vi "ActionSCPICommand.vi"(8 "error in (no error)":errorcluster, 9 "DigitalOuts":T1, 10 "Analogs":T2, 11 "SCPI":string) -> (0 "error out":errorcluster, 3 "OutputMessage":string)   [LabVIEW 2022 SP3]
uses:
  Controls/Analogs.ctl
  Controls/DigitalOuts.ctl
  Controls/DisplayQCommand.ctl
  Controls/DisplayMessage.ctl
  <vilib>/Utility/error.llb/Trim Whitespace One-Sided.vi
  Globals/HandsOnGlobals.vi
panel:
  # "Output"
  # "Input"
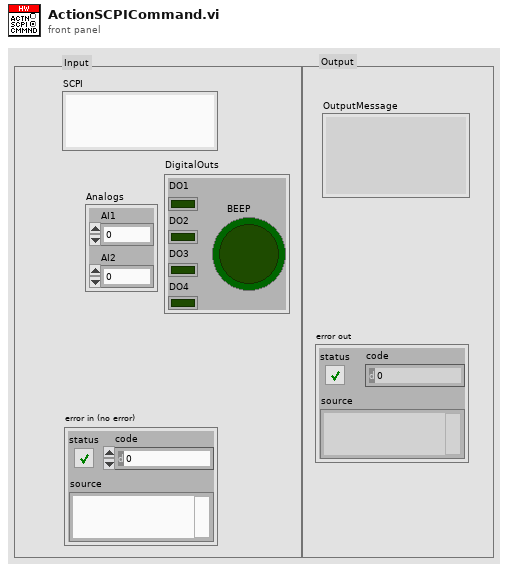
[diagram p1: front panel]
types:
  T1 = typedef "DigitalOuts.ctl" = cluster{"DO1":bool, "DO2":bool, "DO3":bool, "DO4":bool, "BEEP":bool}
  T2 = typedef "Analogs.ctl" = cluster{"AI1":u16, "AI2":u16}
  T3 = typedef "DisplayMessage.ctl" = enum16{"No Message - Ignore", "Display Message", "Set Tab", "Set Status", "Add Error Message", "Clear Error History", "Generate Error", "Set Idling Display", "Set Running Display", "Set DO1", "Set DO2", "Set DO3", "Set DO4", "Set AI1", "Set BEEP", "Update SCPI Return", "Clear SCPI", "Reset Screen", "Set PWM Duty", "Set PWM Freq", "Stop"}
  T4 = typedef "DisplayQCommand.ctl" = enum16{"No Command - Error", "Initialise", "Get Q Reference", "Add Item to Bottom", "Add Item to Top", "Flush Q", "Dequeue", "Peek Next Element", "Close"}
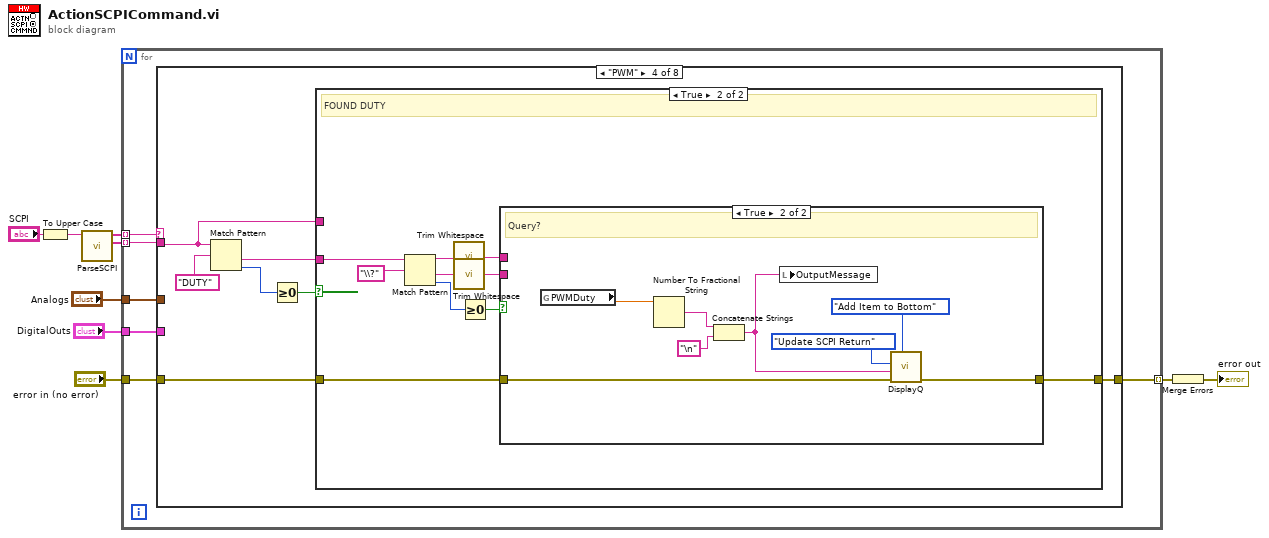
[diagram p0: block diagram]
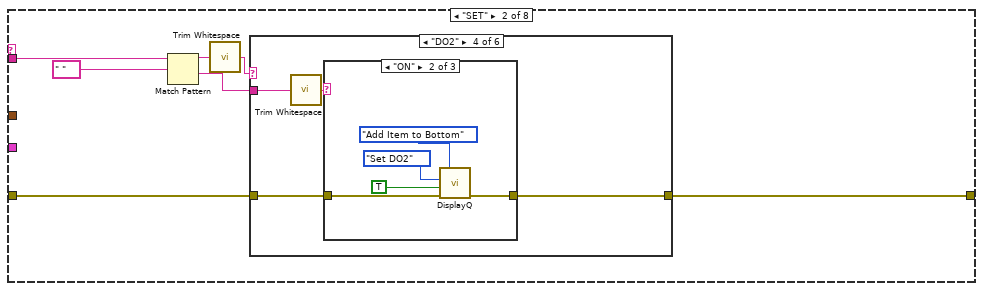
[diagram p3: hidden frame]
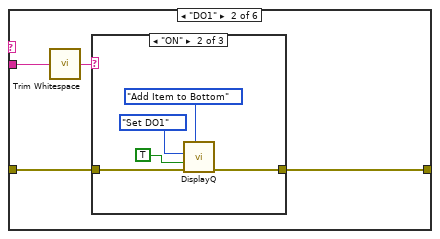
[diagram p5: hidden frame]
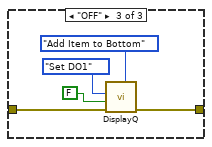
[diagram p7: hidden frame]
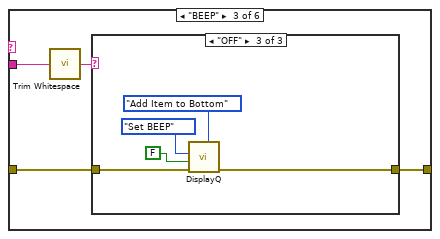
[diagram p8: hidden frame]
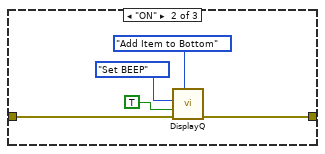
[diagram p10: hidden frame]
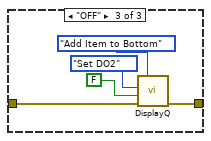
[diagram p12: hidden frame]
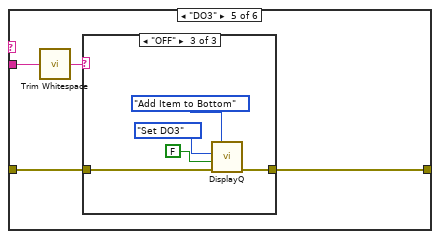
[diagram p13: hidden frame]
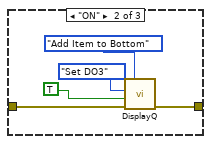
[diagram p15: hidden frame]
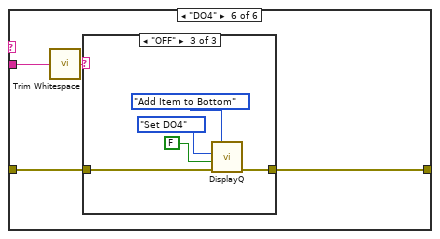
[diagram p16: hidden frame]
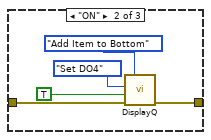
[diagram p18: hidden frame]
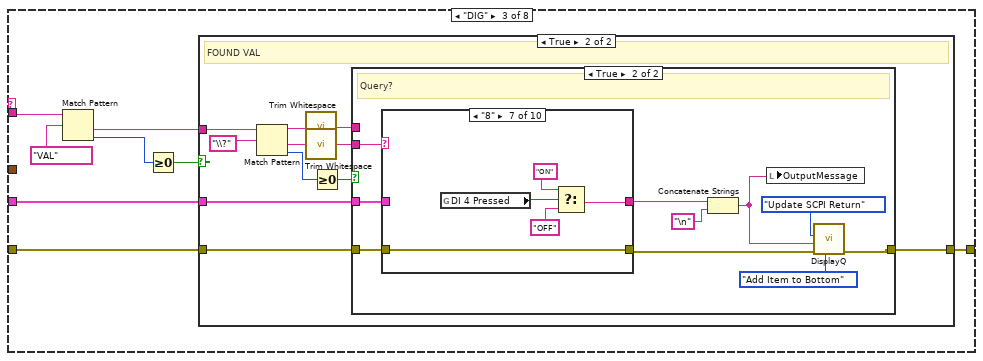
[diagram p19: hidden frame]
diagram:
  n1 = To Upper Case(1:"SCPI") -> (0:w1:string)
  n2 = call "ParseSCPI.vi"("Input String"=w1) -> ("Data Out"=w7:string[], "Commands Out"=w8:string[])  [unwired: 9 in]
  n3 = for {
    tunnel: w8 -> [w15] mode=indexing
    tunnel: w7 -> [w14] mode=indexing
    tunnel: "error in (no error)" -> [w13]
    tunnel: [w12] -> w5 mode=indexing
    tunnel: "Analogs" -> [w11]
    tunnel: "DigitalOuts" -> [w10]
    n4 = case shown="\"PWM\"" w15 {
      tunnel: w14 -> [_ w23 w103 w258 w335 w460 _ _]
      tunnel: w13 -> [w16 w18 w107 w264 w324 w451 w475 w479]
      tunnel: [w16 w17 w106 w263 w329 w456 w477 w481] -> w12
      tunnel: w11 -> [_ _ _ _ w326 w453 _ _]
      tunnel: w10 -> [_ _ w105 _ w325 w452 _ _]
      frame "False", Default {
      }
      frame "SET" {
        n5 = Match Pattern(string=w23, regular expression=" ") -> (before substring=w21:string, after substring=w19:string)  [unwired: 1 in, 2 out]
        n6 = call <vilib>:"Trim Whitespace.vi"("string"=w21) -> ("trimmed string"=w20:string)  [unwired: 1 in]
        n7 = case shown="\"DO2\"" w20 {
          tunnel: w19 -> [_ w28 w43 w58 w73 w88]
          tunnel: w18 -> [w24 w26 w41 w56 w71 w86]
          tunnel: [w24 w25 w40 w55 w70 w85] -> w17
          frame "False", Default {
          }
          frame "DO1" {
            n8 = call <vilib>:"Trim Whitespace.vi"("string"=w28) -> ("trimmed string"=w27:string)  [unwired: 1 in]
            n9 = case shown="\"ON\"" w27 {
              tunnel: w26 -> [w29 w31 w37]
              tunnel: [w29 w32 w36] -> w25
              frame "False", Default {
              }
              frame "ON" {
                n10 = call "DisplayQ.vi"("command"=DisplayQCommand."Add Item to Bottom", "error in (no error)"=w31, "DataIn"=TRUE, "DisplayMessage"=DisplayMessage."Set DO1") -> ("error out"=w32:errorcluster)  [unwired: 1 in, 3 out]
              }
              frame "OFF" {
                n11 = call "DisplayQ.vi"("command"=DisplayQCommand."Add Item to Bottom", "error in (no error)"=w37, "DataIn"=FALSE, "DisplayMessage"=DisplayMessage."Set DO1") -> ("error out"=w36:errorcluster)  [unwired: 1 in, 3 out]
              }
            }
          }
          frame "BEEP" {
            n12 = call <vilib>:"Trim Whitespace.vi"("string"=w43) -> ("trimmed string"=w42:string)  [unwired: 1 in]
            n13 = case shown="\"OFF\"" w42 {
              tunnel: w41 -> [w44 w46 w52]
              tunnel: [w44 w47 w51] -> w40
              frame "False", Default {
              }
              frame "ON" {
                n14 = call "DisplayQ.vi"("command"=DisplayQCommand."Add Item to Bottom", "error in (no error)"=w46, "DataIn"=TRUE, "DisplayMessage"=DisplayMessage."Set BEEP") -> ("error out"=w47:errorcluster)  [unwired: 1 in, 3 out]
              }
              frame "OFF" {
                n15 = call "DisplayQ.vi"("command"=DisplayQCommand."Add Item to Bottom", "error in (no error)"=w52, "DataIn"=FALSE, "DisplayMessage"=DisplayMessage."Set BEEP") -> ("error out"=w51:errorcluster)  [unwired: 1 in, 3 out]
              }
            }
          }
          frame "DO2" {
            n16 = call <vilib>:"Trim Whitespace.vi"("string"=w58) -> ("trimmed string"=w57:string)  [unwired: 1 in]
            n17 = case shown="\"ON\"" w57 {
              tunnel: w56 -> [w59 w61 w67]
              tunnel: [w59 w62 w66] -> w55
              frame "False", Default {
              }
              frame "ON" {
                n18 = call "DisplayQ.vi"("command"=DisplayQCommand."Add Item to Bottom", "error in (no error)"=w61, "DataIn"=TRUE, "DisplayMessage"=DisplayMessage."Set DO2") -> ("error out"=w62:errorcluster)  [unwired: 1 in, 3 out]
              }
              frame "OFF" {
                n19 = call "DisplayQ.vi"("command"=DisplayQCommand."Add Item to Bottom", "error in (no error)"=w67, "DataIn"=FALSE, "DisplayMessage"=DisplayMessage."Set DO2") -> ("error out"=w66:errorcluster)  [unwired: 1 in, 3 out]
              }
            }
          }
          frame "DO3" {
            n20 = call <vilib>:"Trim Whitespace.vi"("string"=w73) -> ("trimmed string"=w72:string)  [unwired: 1 in]
            n21 = case shown="\"OFF\"" w72 {
              tunnel: w71 -> [w74 w76 w82]
              tunnel: [w74 w77 w81] -> w70
              frame "False", Default {
              }
              frame "ON" {
                n22 = call "DisplayQ.vi"("command"=DisplayQCommand."Add Item to Bottom", "error in (no error)"=w76, "DataIn"=TRUE, "DisplayMessage"=DisplayMessage."Set DO3") -> ("error out"=w77:errorcluster)  [unwired: 1 in, 3 out]
              }
              frame "OFF" {
                n23 = call "DisplayQ.vi"("command"=DisplayQCommand."Add Item to Bottom", "error in (no error)"=w82, "DataIn"=FALSE, "DisplayMessage"=DisplayMessage."Set DO3") -> ("error out"=w81:errorcluster)  [unwired: 1 in, 3 out]
              }
            }
          }
          frame "DO4" {
            n24 = call <vilib>:"Trim Whitespace.vi"("string"=w88) -> ("trimmed string"=w87:string)  [unwired: 1 in]
            n25 = case shown="\"OFF\"" w87 {
              tunnel: w86 -> [w89 w91 w97]
              tunnel: [w89 w92 w96] -> w85
              frame "False", Default {
              }
              frame "ON" {
                n26 = call "DisplayQ.vi"("command"=DisplayQCommand."Add Item to Bottom", "error in (no error)"=w91, "DataIn"=TRUE, "DisplayMessage"=DisplayMessage."Set DO4") -> ("error out"=w92:errorcluster)  [unwired: 1 in, 3 out]
              }
              frame "OFF" {
                n27 = call "DisplayQ.vi"("command"=DisplayQCommand."Add Item to Bottom", "error in (no error)"=w97, "DataIn"=FALSE, "DisplayMessage"=DisplayMessage."Set DO4") -> ("error out"=w96:errorcluster)  [unwired: 1 in, 3 out]
              }
            }
          }
        }
      }
      frame "DIG" {
        n28 = Match Pattern(string=w103, regular expression="VAL") -> (after substring=w102:string, offset past match=w101:i32)  [unwired: 1 in, 2 out]
        n29 = Greater Or Equal To 0?(x=w101) -> (x >= 0?=w100:bool)
        n30 = case shown="True" w100 {
          tunnel: w107 -> [w108 w119]
          tunnel: [w108 w118] -> w106
          tunnel: w105 -> [_ w117]
          tunnel: w102 -> [_ w116]
          frame False {
            # "Unrecognised command"
          }
          frame True {
            # "FOUND VAL"
            n31 = Match Pattern(string=w116, regular expression="\\?") -> (before substring=w110:string, after substring=w114:string, offset past match=w112:i32)  [unwired: 1 in, 1 out]
            n32 = call <vilib>:"Trim Whitespace.vi"("string"=w110) -> ("trimmed string"=w109:string)  [unwired: 1 in]
            n33 = call <vilib>:"Trim Whitespace.vi"("string"=w114) -> ("trimmed string"=w113:string)  [unwired: 1 in]
            n34 = Greater Or Equal To 0?(x=w112) -> (x >= 0?=w111:bool)
            n35 = case shown="True" w111 {
              tunnel: w119 -> [w125 w206]
              tunnel: [w124 w199] -> w118
              tunnel: w117 -> [_ w205]
              tunnel: w113 -> [_ w204]
              tunnel: w109 -> [w120 _]
              frame False {
                # "Set"
                n36 = Match Pattern(string=w120, regular expression=",") -> (before substring=w121:string, after substring=w122:string)  [unwired: 1 in, 2 out]
                n37 = case shown="\"0\"" w121 {
                  tunnel: w125 -> [w126 w129 w143 w157 w171 w185]
                  tunnel: [w126 w128 w142 w156 w170 w184] -> w124
                  tunnel: w122 -> [_ w127 w141 w155 w169 w183]
                  frame "False", Default {
                  }
                  frame "0" {
                    n38 = case shown="\"1\"" w127 {
                      tunnel: w129 -> [w130 w132 w138]
                      tunnel: [w130 w133 w137] -> w128
                      frame "False", Default {
                      }
                      frame "1" {
                        n39 = call "DisplayQ.vi"("command"=DisplayQCommand."Add Item to Bottom", "error in (no error)"=w132, "DataIn"=TRUE, "DisplayMessage"=DisplayMessage."Set DO1") -> ("error out"=w133:errorcluster)  [unwired: 1 in, 3 out]
                      }
                      frame "0" {
                        n40 = call "DisplayQ.vi"("command"=DisplayQCommand."Add Item to Bottom", "error in (no error)"=w138, "DataIn"=FALSE, "DisplayMessage"=DisplayMessage."Set DO1") -> ("error out"=w137:errorcluster)  [unwired: 1 in, 3 out]
                      }
                    }
                  }
                  frame "1" {
                    n41 = case shown="\"1\"" w141 {
                      tunnel: w143 -> [w144 w146 w152]
                      tunnel: [w144 w147 w151] -> w142
                      frame "False", Default {
                      }
                      frame "1" {
                        n42 = call "DisplayQ.vi"("command"=DisplayQCommand."Add Item to Bottom", "error in (no error)"=w146, "DataIn"=TRUE, "DisplayMessage"=DisplayMessage."Set DO2") -> ("error out"=w147:errorcluster)  [unwired: 1 in, 3 out]
                      }
                      frame "0" {
                        n43 = call "DisplayQ.vi"("command"=DisplayQCommand."Add Item to Bottom", "error in (no error)"=w152, "DataIn"=FALSE, "DisplayMessage"=DisplayMessage."Set DO2") -> ("error out"=w151:errorcluster)  [unwired: 1 in, 3 out]
                      }
                    }
                  }
                  frame "2" {
                    n44 = case shown="\"1\"" w155 {
                      tunnel: w157 -> [w158 w160 w166]
                      tunnel: [w158 w161 w165] -> w156
                      frame "False", Default {
                      }
                      frame "1" {
                        n45 = call "DisplayQ.vi"("command"=DisplayQCommand."Add Item to Bottom", "error in (no error)"=w160, "DataIn"=TRUE, "DisplayMessage"=DisplayMessage."Set DO3") -> ("error out"=w161:errorcluster)  [unwired: 1 in, 3 out]
                      }
                      frame "0" {
                        n46 = call "DisplayQ.vi"("command"=DisplayQCommand."Add Item to Bottom", "error in (no error)"=w166, "DataIn"=FALSE, "DisplayMessage"=DisplayMessage."Set DO3") -> ("error out"=w165:errorcluster)  [unwired: 1 in, 3 out]
                      }
                    }
                  }
                  frame "3" {
                    n47 = case shown="\"1\"" w169 {
                      tunnel: w171 -> [w172 w174 w180]
                      tunnel: [w172 w175 w179] -> w170
                      frame "False", Default {
                      }
                      frame "1" {
                        n48 = call "DisplayQ.vi"("command"=DisplayQCommand."Add Item to Bottom", "error in (no error)"=w174, "DataIn"=TRUE, "DisplayMessage"=DisplayMessage."Set DO4") -> ("error out"=w175:errorcluster)  [unwired: 1 in, 3 out]
                      }
                      frame "0" {
                        n49 = call "DisplayQ.vi"("command"=DisplayQCommand."Add Item to Bottom", "error in (no error)"=w180, "DataIn"=FALSE, "DisplayMessage"=DisplayMessage."Set DO4") -> ("error out"=w179:errorcluster)  [unwired: 1 in, 3 out]
                      }
                    }
                  }
                  frame "4" {
                    n50 = case shown="\"1\"" w183 {
                      tunnel: w185 -> [w186 w188 w194]
                      tunnel: [w186 w189 w193] -> w184
                      frame "False", Default {
                      }
                      frame "1" {
                        n51 = call "DisplayQ.vi"("command"=DisplayQCommand."Add Item to Bottom", "error in (no error)"=w188, "DataIn"=TRUE, "DisplayMessage"=DisplayMessage."Set BEEP") -> ("error out"=w189:errorcluster)  [unwired: 1 in, 3 out]
                      }
                      frame "0" {
                        n52 = call "DisplayQ.vi"("command"=DisplayQCommand."Add Item to Bottom", "error in (no error)"=w194, "DataIn"=FALSE, "DisplayMessage"=DisplayMessage."Set BEEP") -> ("error out"=w193:errorcluster)  [unwired: 1 in, 3 out]
                      }
                    }
                  }
                }
              }
              frame True {
                # "Query?"
                n53 = case shown="\"8\"" w204 {
                  tunnel: [w207 w210 w216 w222 w227 w232 w237 w243 w249 w255] -> w198
                  tunnel: [_ w208 w214 w221 w226 w231 w236 w240 w246 w252] -> w197
                  tunnel: w206 -> [w207 w210 w216 w222 w227 w232 w237 w243 w249 w255]
                  tunnel: w205 -> [_ w209 w215 _ _ _ _ w241 w247 w253]
                  frame "False", Default {
                  }
                  frame "0" {
                    n54 = Unbundle By Name(w209) -> ("DO1"=w212:bool)
                    n55 = Select(t="ON", s=w212, f="OFF") -> (s? t:f=w208:string)
                  }
                  frame "4" {
                    n56 = Unbundle By Name(w215) -> ("BEEP"=w218:bool)
                    n57 = Select(t="ON", s=w218, f="OFF") -> (s? t:f=w214:string)
                  }
                  frame "5" {
                    n58 = global read "HandsOnGlobals.vi" "DI 1 Pressed"() -> (w220:bool)
                    n59 = Select(t="ON", s=w220, f="OFF") -> (s? t:f=w221:string)
                  }
                  frame "6" {
                    n60 = global read "HandsOnGlobals.vi" "DI 2 Pressed"() -> (w225:bool)
                    n61 = Select(t="ON", s=w225, f="OFF") -> (s? t:f=w226:string)
                  }
                  frame "7" {
                    n62 = global read "HandsOnGlobals.vi" "DI 3 Pressed"() -> (w230:bool)
                    n63 = Select(t="ON", s=w230, f="OFF") -> (s? t:f=w231:string)
                  }
                  frame "8" {
                    n64 = global read "HandsOnGlobals.vi" "DI 4 Pressed"() -> (w235:bool)
                    n65 = Select(t="ON", s=w235, f="OFF") -> (s? t:f=w236:string)
                  }
                  frame "1" {
                    n66 = Unbundle By Name(w241) -> ("DO2"=w244:bool)
                    n67 = Select(t="ON", s=w244, f="OFF") -> (s? t:f=w240:string)
                  }
                  frame "2" {
                    n68 = Unbundle By Name(w247) -> ("DO3"=w250:bool)
                    n69 = Select(t="ON", s=w250, f="OFF") -> (s? t:f=w246:string)
                  }
                  frame "3" {
                    n70 = Unbundle By Name(w253) -> ("DO4"=w256:bool)
                    n71 = Select(t="ON", s=w256, f="OFF") -> (s? t:f=w252:string)
                  }
                }
                n72 = Concatenate Strings(w197, "\n" ("string")) -> (w203:string)
                n73 = local write "OutputMessage"(w203) -> ()
                n74 = call "DisplayQ.vi"("command"=DisplayQCommand."Add Item to Bottom", "error in (no error)"=w198, "DataIn"=w203, "DisplayMessage"=DisplayMessage."Update SCPI Return") -> ("error out"=w199:errorcluster)  [unwired: 1 in, 3 out]
              }
            }
          }
        }
      }
      frame "PWM" {
        n75 = Match Pattern(string=w258, regular expression="DUTY") -> (after substring=w261:string, offset past match=w260:i32)  [unwired: 1 in, 2 out]
        n76 = Greater Or Equal To 0?(x=w260) -> (x >= 0?=w259:bool)
        n77 = case shown="True" w259 {
          tunnel: w264 -> [w271 w307]
          tunnel: [w270 w306] -> w263
          tunnel: w261 -> [_ w305]
          tunnel: w258 -> [w268 _]
          frame False {
            # "Unrecognised command"
            n78 = Match Pattern(string=w268, regular expression="FREQ") -> (after substring=w265:string, offset past match=w267:i32)  [unwired: 1 in, 2 out]
            n79 = Greater Or Equal To 0?(x=w267) -> (x >= 0?=w266:bool)
            n80 = case shown="True" w266 {
              tunnel: w271 -> [w272 w275]
              tunnel: [w272 w274] -> w270
              tunnel: w265 -> [_ w273]
              frame False {
                # "Unrecognised command"
              }
              frame True {
                # "FOUND FREQ"
                n81 = Match Pattern(string=w273, regular expression="\\?") -> (before substring=w277:string, after substring=w281:string, offset past match=w279:i32)  [unwired: 1 in, 1 out]
                n82 = call <vilib>:"Trim Whitespace.vi"("string"=w277) -> ("trimmed string"=w276:string)  [unwired: 1 in]
                n83 = call <vilib>:"Trim Whitespace.vi"("string"=w281) -> ("trimmed string"=w280:string)  [unwired: 1 in]
                n84 = Greater Or Equal To 0?(x=w279) -> (x >= 0?=w278:bool)
                n85 = case shown="True" w278 {
                  tunnel: w275 -> [w289 w293]
                  tunnel: [w288 w292] -> w274
                  tunnel: w280 -> [_ _]
                  tunnel: w276 -> [w285 _]
                  frame False {
                    # "Set"
                    n86 = Scan From String(format string="%f,%f", input string=w285) -> (output 2=w283:dbl)  [unwired: 5 in, 3 out]
                    n87 = call "DisplayQ.vi"("command"=DisplayQCommand."Add Item to Bottom", "error in (no error)"=w289, "DataIn"=w283, "DisplayMessage"=DisplayMessage."Set PWM Freq") -> ("error out"=w288:errorcluster)  [unwired: 1 in, 3 out]
                  }
                  frame True {
                    # "Query?"
                    n88 = global read "HandsOnGlobals.vi" "PWMFreq"() -> (w291:dbl)
                    n89 = Number To Fractional String(number=w291) -> (F-format string=w294:string)  [unwired: 3 in]
                    n90 = Concatenate Strings(w294, "\n" ("string")) -> (w290:string)
                    n91 = local write "OutputMessage"(w290) -> ()
                    n92 = call "DisplayQ.vi"("command"=DisplayQCommand."Add Item to Bottom", "error in (no error)"=w293, "DataIn"=w290, "DisplayMessage"=DisplayMessage."Update SCPI Return") -> ("error out"=w292:errorcluster)  [unwired: 1 in, 3 out]
                  }
                }
              }
            }
          }
          frame True {
            # "FOUND DUTY"
            n93 = Match Pattern(string=w305, regular expression="\\?") -> (before substring=w299:string, after substring=w303:string, offset past match=w301:i32)  [unwired: 1 in, 1 out]
            n94 = call <vilib>:"Trim Whitespace.vi"("string"=w299) -> ("trimmed string"=w298:string)  [unwired: 1 in]
            n95 = call <vilib>:"Trim Whitespace.vi"("string"=w303) -> ("trimmed string"=w302:string)  [unwired: 1 in]
            n96 = Greater Or Equal To 0?(x=w301) -> (x >= 0?=w300:bool)
            n97 = case shown="True" w300 {
              tunnel: w307 -> [w314 w319]
              tunnel: [w313 w320] -> w306
              tunnel: w302 -> [_ _]
              tunnel: w298 -> [w310 _]
              frame False {
                # "Set"
                n98 = Scan From String(format string="%f,%f", input string=w310) -> (output 2=w308:dbl)  [unwired: 5 in, 3 out]
                n99 = call "DisplayQ.vi"("command"=DisplayQCommand."Add Item to Bottom", "error in (no error)"=w314, "DataIn"=w308, "DisplayMessage"=DisplayMessage."Set PWM Duty") -> ("error out"=w313:errorcluster)  [unwired: 1 in, 3 out]
              }
              frame True {
                # "Query?"
                n100 = global read "HandsOnGlobals.vi" "PWMDuty"() -> (w318:dbl)
                n101 = Number To Fractional String(number=w318) -> (F-format string=w316:string)  [unwired: 3 in]
                n102 = Concatenate Strings(w316, "\n" ("string")) -> (w315:string)
                n103 = local write "OutputMessage"(w315) -> ()
                n104 = call "DisplayQ.vi"("command"=DisplayQCommand."Add Item to Bottom", "error in (no error)"=w319, "DataIn"=w315, "DisplayMessage"=DisplayMessage."Update SCPI Return") -> ("error out"=w320:errorcluster)  [unwired: 1 in, 3 out]
              }
            }
          }
        }
      }
      frame "GET" {
        n105 = Match Pattern(string=w335, regular expression=":") -> (before substring=w333:string, after substring=w331:string)  [unwired: 1 in, 2 out]
        n106 = call <vilib>:"Trim Whitespace.vi"("string"=w333) -> ("trimmed string"=w332:string)  [unwired: 1 in]
        n107 = case shown="\"DO1?\"" w332 {
          tunnel: w331 -> [_ _ _ _ _ _ _ _ _ _ _ _]
          tunnel: [w336 w338 w346 w353 w372 w377 w378 w393 w408 w426 w432 w440] -> w327
          tunnel: [_ w337 w345 w357 w370 w375 w382 w397 w412 w424 w433 w441] -> w323
          tunnel: w326 -> [_ _ _ _ w371 w376 _ _ _ _ _ _]
          tunnel: w325 -> [_ w339 w347 _ _ _ _ _ _ w425 w434 w442]
          tunnel: w324 -> [w336 w338 w346 w354 w372 w377 w379 w394 w409 w426 w432 w440]
          frame "False", Default {
          }
          frame "DO1?" {
            n108 = Unbundle By Name(w339) -> ("DO1"=w341:bool)
            n109 = Select(t="ON", s=w341, f="OFF") -> (s? t:f=w343:string)
            n110 = Concatenate Strings("DO1 ", w343) -> (w337:string)
          }
          frame "BEEP?" {
            n111 = Unbundle By Name(w347) -> ("BEEP"=w349:bool)
            n112 = Select(t="ON", s=w349, f="OFF") -> (s? t:f=w351:string)
            n113 = Concatenate Strings("BEEP ", w351) -> (w345:string)
          }
          frame "DI1?" {
            n114 = flat-sequence {
              tunnel: [w359] -> w356
              tunnel: [w358] -> w355
              tunnel: w354 -> [w358]
              tunnel: [w367] -> w357
              tunnel: w356 -> [w367]
              tunnel: [w365] -> w353
              tunnel: w355 -> [w365]
              frame #0 {
                n115 = global read "HandsOnGlobals.vi" "DI 1 Pressed"() -> (w364:bool)
                n116 = Select(t="ON", s=w364, f="OFF") -> (s? t:f=w361:string)
                n117 = Concatenate Strings("DI1 ", w361) -> (w359:string)
              }
              frame #1 {
                n118 = global write "HandsOnGlobals.vi" "DI 1 Pressed"(FALSE ("DI 1 Pressed")) -> ()
              }
            }
          }
          frame "AI1?" {
            w369 = TRUE  # use system decimal point (T)
            n119 = Unbundle By Name(w371) -> ("AI1"=w368:u16)
            n120 = Number To Fractional String(use system decimal point (T)=w369, number=w368) -> (F-format string=w370:string)  [unwired: 2 in]
          }
          frame "AI2?" {
            w374 = TRUE  # use system decimal point (T)
            n121 = Unbundle By Name(w376) -> ("AI2"=w373:u16)
            n122 = Number To Fractional String(use system decimal point (T)=w374, number=w373) -> (F-format string=w375:string)  [unwired: 2 in]
          }
          frame "DI2?" {
            n123 = flat-sequence {
              tunnel: [w384] -> w381
              tunnel: [w383] -> w380
              tunnel: w379 -> [w383]
              tunnel: [w392] -> w382
              tunnel: w381 -> [w392]
              tunnel: [w390] -> w378
              tunnel: w380 -> [w390]
              frame #0 {
                n124 = global read "HandsOnGlobals.vi" "DI 2 Pressed"() -> (w389:bool)
                n125 = Select(t="ON", s=w389, f="OFF") -> (s? t:f=w386:string)
                n126 = Concatenate Strings("DI2 ", w386) -> (w384:string)
              }
              frame #1 {
                n127 = global write "HandsOnGlobals.vi" "DI 2 Pressed"(FALSE ("DI 1 Pressed")) -> ()
              }
            }
          }
          frame "DI3?" {
            n128 = flat-sequence {
              tunnel: [w399] -> w396
              tunnel: [w398] -> w395
              tunnel: w394 -> [w398]
              tunnel: [w407] -> w397
              tunnel: w396 -> [w407]
              tunnel: [w405] -> w393
              tunnel: w395 -> [w405]
              frame #0 {
                n129 = global read "HandsOnGlobals.vi" "DI 3 Pressed"() -> (w404:bool)
                n130 = Select(t="ON", s=w404, f="OFF") -> (s? t:f=w401:string)
                n131 = Concatenate Strings("DI3 ", w401) -> (w399:string)
              }
              frame #1 {
                n132 = global write "HandsOnGlobals.vi" "DI 3 Pressed"(FALSE ("DI 1 Pressed")) -> ()
              }
            }
          }
          frame "DI4?" {
            n133 = flat-sequence {
              tunnel: [w414] -> w411
              tunnel: [w413] -> w410
              tunnel: w409 -> [w413]
              tunnel: [w422] -> w412
              tunnel: w411 -> [w422]
              tunnel: [w420] -> w408
              tunnel: w410 -> [w420]
              frame #0 {
                n134 = global read "HandsOnGlobals.vi" "DI 4 Pressed"() -> (w419:bool)
                n135 = Select(t="ON", s=w419, f="OFF") -> (s? t:f=w416:string)
                n136 = Concatenate Strings("DI4 ", w416) -> (w414:string)
              }
              frame #1 {
                n137 = global write "HandsOnGlobals.vi" "DI 4 Pressed"(FALSE ("DI 1 Pressed")) -> ()
              }
            }
          }
          frame "DO2?" {
            n138 = Unbundle By Name(w425) -> ("DO2"=w427:bool)
            n139 = Select(t="ON", s=w427, f="OFF") -> (s? t:f=w429:string)
            n140 = Concatenate Strings("DO2 ", w429) -> (w424:string)
          }
          frame "DO3?" {
            n141 = Unbundle By Name(w434) -> ("DO3"=w435:bool)
            n142 = Select(t="ON", s=w435, f="OFF") -> (s? t:f=w437:string)
            n143 = Concatenate Strings("DO3 ", w437) -> (w433:string)
          }
          frame "DO4?" {
            n144 = Unbundle By Name(w442) -> ("DO4"=w443:bool)
            n145 = Select(t="ON", s=w443, f="OFF") -> (s? t:f=w445:string)
            n146 = Concatenate Strings("DO4 ", w445) -> (w441:string)
          }
        }
        "OutputMessage" <- w323
        n147 = call "DisplayQ.vi"("command"=DisplayQCommand."Add Item to Bottom", "error in (no error)"=w327, "DataIn"=w323, "DisplayMessage"=DisplayMessage."Update SCPI Return") -> ("error out"=w329:errorcluster)  [unwired: 1 in, 3 out]
      }
      frame "ANA" {
        n148 = Match Pattern(string=w460, regular expression="VAL\\? ") -> (after substring=w450:string)  [unwired: 1 in, 3 out]
        n149 = call <vilib>:"Trim Whitespace.vi"("string"=w450) -> ("trimmed string"=w458:string)  [unwired: 1 in]
        n150 = case shown="\"2\"" w458 {
          tunnel: [w461 w465 w469] -> w454
          tunnel: [_ w463 w466] -> w448
          tunnel: w453 -> [_ w464 w468]
          tunnel: w452 -> [_ _ _]
          tunnel: w451 -> [w461 w465 w469]
          frame "False", Default {
          }
          frame "1" {
            n151 = Unbundle By Name(w464) -> ("AI1"=w462:u16)
            n152 = Number To Decimal String(number=w462) -> (decimal integer string=w463:string)  [unwired: 1 in]
          }
          frame "2" {
            n153 = Unbundle By Name(w468) -> ("AI2"=w467:u16)
            n154 = Number To Decimal String(number=w467) -> (decimal integer string=w466:string)  [unwired: 1 in]
          }
        }
        n155 = Concatenate Strings(w448, "\n" ("string")) -> (w447:string)
        n156 = local write "OutputMessage"(w447) -> ()
        n157 = call "DisplayQ.vi"("command"=DisplayQCommand."Add Item to Bottom", "error in (no error)"=w454, "DataIn"=w447, "DisplayMessage"=DisplayMessage."Update SCPI Return") -> ("error out"=w456:errorcluster)  [unwired: 1 in, 3 out]
      }
      frame "*IDN?" {
        n158 = call "Version.vi"() -> ("Version"=w474:string)  [unwired: 5 in]
        n159 = Format Into String(format string="CTI,RP2040-Visa,Emulator,%s20230827T193959Z" ("data in"), w474) -> (resulting string=w471:string)  [unwired: 2 in, 1 out]
        n160 = Concatenate Strings(w471, "\n" ("string")) -> (w470:string)
        n161 = local write "OutputMessage"(w470) -> ()
        n162 = call "DisplayQ.vi"("command"=DisplayQCommand."Add Item to Bottom", "error in (no error)"=w475, "DataIn"=w470, "DisplayMessage"=DisplayMessage."Update SCPI Return") -> ("error out"=w477:errorcluster)  [unwired: 1 in, 3 out]
      }
      frame "*RST" {
        n163 = call "DisplayQ.vi"("command"=DisplayQCommand."Add Item to Bottom", "error in (no error)"=w479, "DisplayMessage"=DisplayMessage."Reset Screen") -> ("error out"=w481:errorcluster)  [unwired: 2 in, 3 out]
      }
    }
  }
  n164 = Merge Errors(w5) -> (→"error out":errorcluster)
